vi "lab1-1.vi"() -> ()   [LabVIEW 2015]
panel:
  out "Boolean":bool
  in  "Numeric":dbl
  out "Thermometer":dbl(slide) scale=0.0..100.0
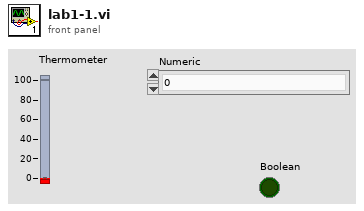
[diagram p1: front panel]
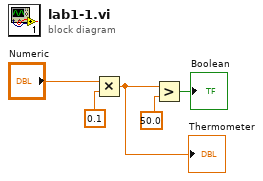
[diagram p0: block diagram]
diagram:
  n1 = Multiply(x="Numeric", y=0.1) -> (x*y=w2:dbl)
  "Thermometer" <- w2
  n2 = Greater?(x=w2, y=50.0) -> (0:→"Boolean":bool)
